vi "Get UUT Serial Port Parameters.vi"(0 "VISA resource name":refnum<visa-resource-name>, 11 "error in (no error)":errorcluster) -> (3 "Baud Rate":i32, 4 "VISA resource name out":refnum<visa-resource-name>, 6 "Flow Control":i32, 8 "Number Data Bits":i32, 10 "Number Stop Bits":i32, 14 "Parity":i32, 15 "error out":errorcluster)   [LabVIEW 2014, in "Fluke 5XXX Series Multicalibrators.lvlib"]
doc: "This VI returns the RS-232-C settings for the Calibrator rear panel SERIAL 2 TO UUT serial port.\n\nNote:\n\nThis VI is available only for instrument models 5500A and 5520A."
uses:
  Fluke 5XXX Series Multicalibrators.lvlib
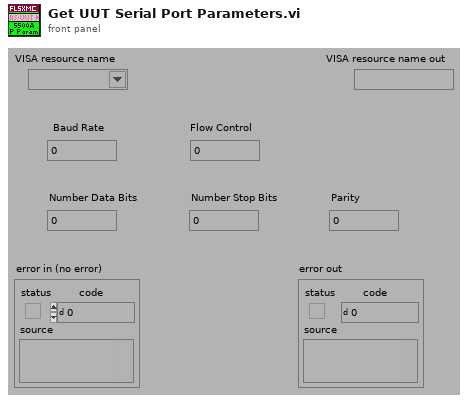
[diagram p1: front panel]
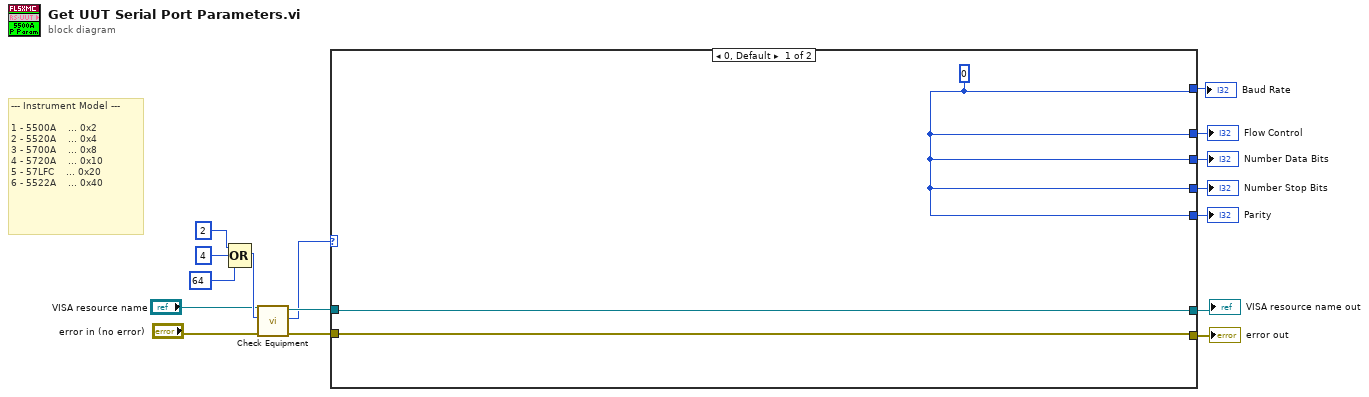
[diagram p0: block diagram]
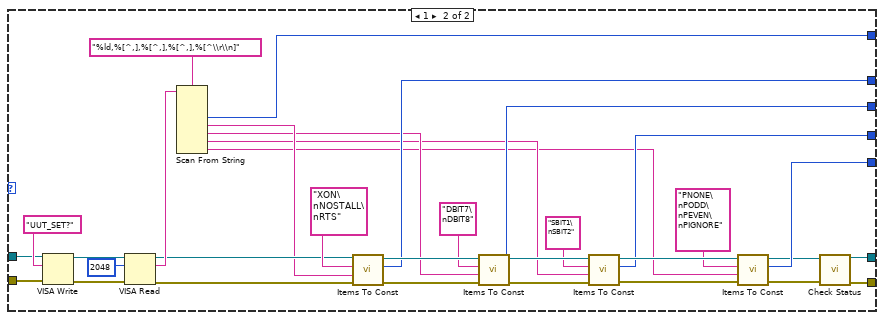
[diagram p2: hidden frame]
diagram:
  # "--- Instrument Model ---\n\n1 - 5500A    ... 0x2\n2 - 5520A    ... 0x4\n3 - 5700A    ... 0x8\n4 - 5720A    ... 0x10\n5 - 57LFC    ... 0x20\n6 - 5522A    ... 0x40"
  n1 = Compound Arithmetic op=OR(2 ("Numeric"), 4 ("Numeric"), 64 ("Numeric")) -> (w12:i32)
  n2 = call "Check Equipment.vi"("error in (no error)"="error in (no error)", "Bit Mask"=w12, "VISA resource name"="VISA resource name") -> ("error out"=w10:errorcluster, "Present?"=w7:u32, "VISA resource name out"=w8:refnum<visa-resource-name>)  [unwired: 6 in]
  n3 = case shown="0, Default" w7 {
    tunnel: [w19 w36] -> w16
    tunnel: [w18 w35] -> w15
    tunnel: w10 -> [w19 w34]
    tunnel: w8 -> [w18 w33]
    tunnel: [w17 w32] -> w6
    tunnel: [w17 w31] -> w5
    tunnel: [w17 w30] -> w4
    tunnel: [w17 w29] -> w3
    tunnel: [w17 w28] -> w2
    frame 0, Default {
      w17 = 0
    }
    frame 1 {
      n4 = VISA Write(VISA resource name=w33, write buffer="UUT_SET?", error in (no error)=w34) -> (VISA resource name out=w51:refnum<visa-resource-name>, error out=w50:errorcluster)  [unwired: 1 out]
      n5 = VISA Read(VISA resource name=w51, byte count=u32 2048 ("byte count (0)"), error in (no error)=w50) -> (VISA resource name out=w25:refnum<visa-resource-name>, read buffer=w47:string, error out=w24:errorcluster)  [unwired: 1 out]
      n6 = Scan From String(format string="%ld,%[^,],%[^,],%[^,],%[^\\r\\n]", input string=w47) -> (output 1=w32:i32, output 2=w23:string, output 3=w22:string, output 4=w21:string, output 5=w20:string)  [unwired: 7 in, 3 out]
      n7 = call "Items To Const.vi"("error in (no error)"=w24, "String Item"=w23, "Multi-Line String"="XON\nNOSTALL\nRTS" ("Reset Command"), "VISA resource name"=w25) -> ("error out"=w46:errorcluster, "Index"=w31:i32, "VISA resource name out"=w43:refnum<visa-resource-name>)  [unwired: 5 in]
      n8 = call "Items To Const.vi"("error in (no error)"=w46, "String Item"=w22, "Multi-Line String"="DBIT7\nDBIT8" ("Reset Command"), "VISA resource name"=w43) -> ("error out"=w45:errorcluster, "Index"=w30:i32, "VISA resource name out"=w42:refnum<visa-resource-name>)  [unwired: 5 in]
      n9 = call "Items To Const.vi"("error in (no error)"=w45, "String Item"=w21, "Multi-Line String"="SBIT1\nSBIT2" ("Reset Command"), "VISA resource name"=w42) -> ("error out"=w44:errorcluster, "Index"=w29:i32, "VISA resource name out"=w41:refnum<visa-resource-name>)  [unwired: 5 in]
      n10 = call "Items To Const.vi"("error in (no error)"=w44, "String Item"=w20, "Multi-Line String"="PNONE\nPODD\nPEVEN\nPIGNORE" ("Reset Command"), "VISA resource name"=w41) -> ("error out"=w27:errorcluster, "Index"=w28:i32, "VISA resource name out"=w26:refnum<visa-resource-name>)  [unwired: 5 in]
      n11 = call "Check Status.vi"("VISA resource name"=w26, "error in (no error)"=w27) -> ("VISA resource name out"=w35:refnum<visa-resource-name>, "error out"=w36:errorcluster)  [unwired: 12 in]
    }
  }
  "Baud Rate" <- w6
  "Flow Control" <- w5
  "Number Data Bits" <- w4
  "Number Stop Bits" <- w3
  "Parity" <- w2
  "VISA resource name out" <- w15
  "error out" <- w16
